vi "Init ADC.vi"(8 "error in (no error)":errorcluster, 11 "NAU7802 in":refnum<class "Adafruit NAU7802 24bit Strain Gauge.lvclass">) -> (0 "error out":errorcluster, 3 "NAU7802 out":refnum<class "Adafruit NAU7802 24bit Strain Gauge.lvclass">)   [LabVIEW 2020, in "CTI-Peripheral.lvlib" / "Adafruit NAU7802 24bit Strain Gauge.lvclass"]
uses:
  Adafruit NAU7802 24bit Strain Gauge.lvclass
  Adafruit NAU7802 24bit Strain Gauge.lvclass/Adafruit NAU7802 24bit Strain Gauge.ctl
  CTI/I2C Connection/I2C Connection.lvclass/I2C Connection.ctl
  bd0b86fe-fbb3-4e34-a7fd-dc47f320ece8.vi
  CTI/Session/I2C Write Data.vi
  CTI/I2C Connection/I2C Connection.lvclass
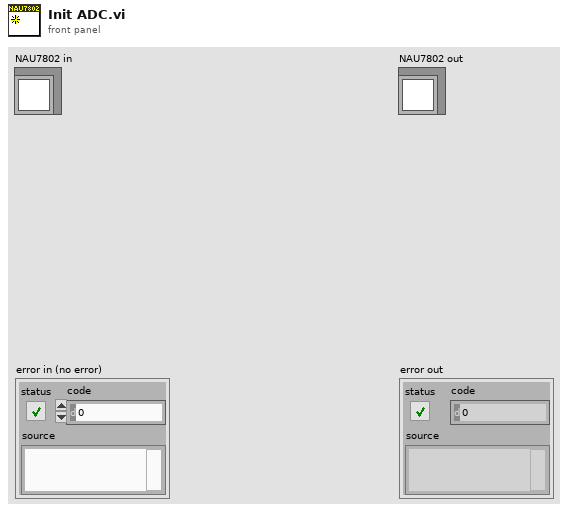
[diagram p1: front panel]
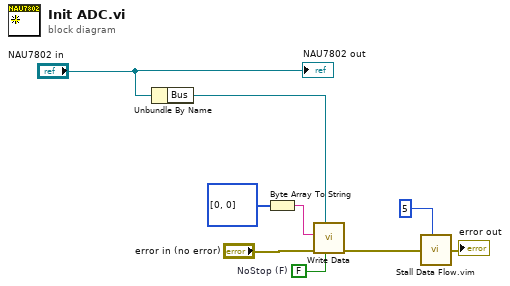
[diagram p0: block diagram]
diagram:
  w6 = FALSE  # NoStop (F)
  n1 = Unbundle By Name("NAU7802 in") -> ("Bus"=w8:refnum<class "I2C Connection.lvclass">)
  n2 = Byte Array To String(unsigned byte array=u8[] [0, 0]) -> (string=w5:string)
  n3 = call "Write Data.vi"("NoStop (F)"=w6, "I2C Connection"=w8, "error in (no error)"="error in (no error)", "Data"=w5) -> ("error out"=w3:errorcluster)  [unwired: 7 in]
  n4 = call "Stall Data Flow.vim"("value in"=w3, "milliseconds to wait"=u32 5) -> ("value out"=→"error out":errorcluster)  [unwired: 1 out]
  "NAU7802 out" <- "NAU7802 in"
